vi "AddVIsToDictionary.vi"(7 "VIs in":refnum<vi>[](array[refnum]), 8 "error in (no error)":errorcluster, 11 "Dictionary from File":T1) -> (0 "error out":errorcluster, 3 "Merged Dictionary":T1)   [LabVIEW 2017, in "JKI Simple Localization.lvlib"]
uses:
  API/JKI Simple Localization.lvlib
  Definitions/Dictionary--Cluster.ctl
  Definitions/Private/FontCluster.ctl
  Definitions/Private/Phrase Dictionary.ctl
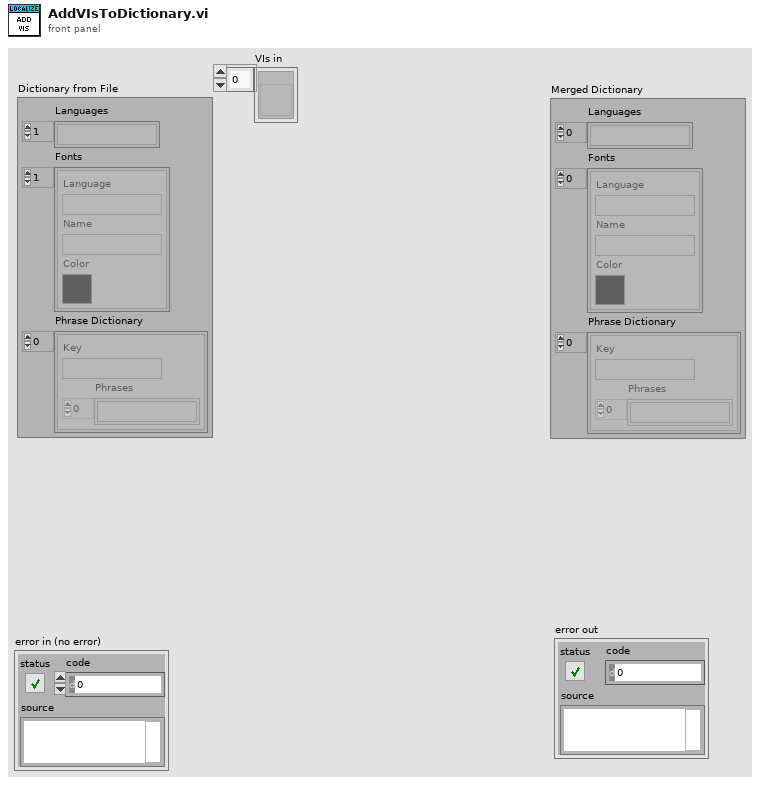
[diagram p1: front panel]
types:
  T1 = typedef "JKI Simple Localization.lvlib/Dictionary--Cluster.ctl" = cluster{"Languages":string[], "Fonts":T2[], "Phrase Dictionary":T3[]}
  T2 = typedef "JKI Simple Localization.lvlib/FontCluster.ctl" = cluster{"Language":string, "Name":string, "Color":u32}
  T3 = typedef "JKI Simple Localization.lvlib/Phrase Dictionary.ctl" = cluster{"Key":string, "Phrases":string[]}
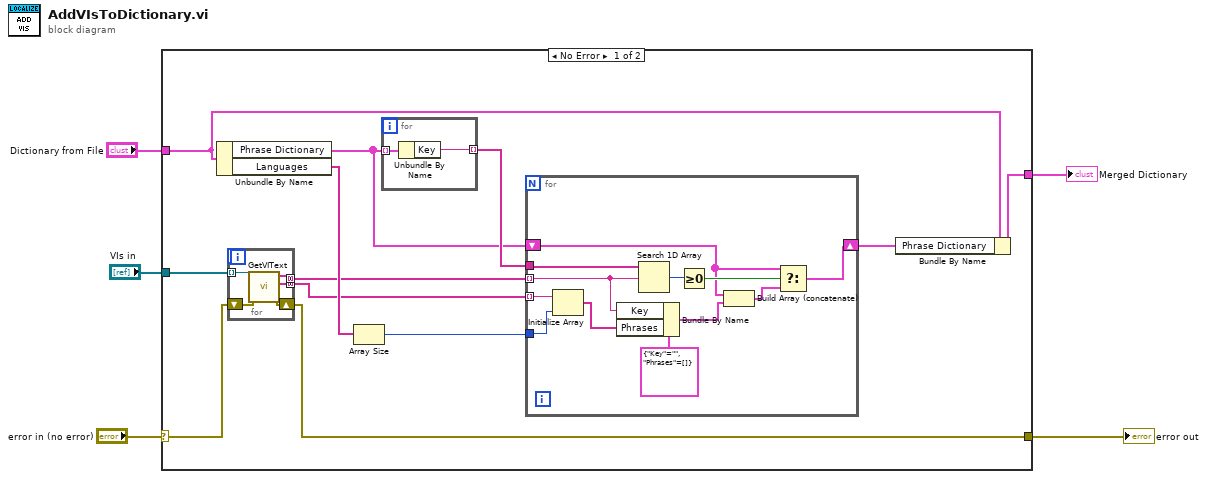
[diagram p0: block diagram]
diagram:
  n1 = case shown="No Error" "error in (no error)" {
    selector: "error in (no error)" -> [w14 w38]
    tunnel: [w13 w38] -> w4
    tunnel: "Dictionary from File" -> [w16 w37]
    tunnel: [w17 w37] -> w2
    tunnel: "VIs in" -> [w15 _]
    frame No Error {
      n2 = Unbundle By Name(w16) -> ("Phrase Dictionary"=w11:T3[], "Languages"=w10:string[])
      n3 = for {
        tunnel: [w22] -> w6 mode=concatenating
        tunnel: [w21] -> w7 mode=concatenating
        shift-right: [w20] -> w13
        shift-left: w14 -> [w19]
        tunnel: w15 -> [w18] mode=indexing
        n4 = call "GetVIText.vi"("error in (no error)"=w19, "VI"=w18) -> ("error out"=w20:errorcluster, "Control Text"=w22:string[], "Control Keys"=w21:string[])  [unwired: 7 in]
      }
      n5 = Array Size(array=w10) -> (size(s)=w9:i32)
      n6 = for {
        tunnel: w11 -> [w24] mode=indexing
        tunnel: [w23] -> w12 mode=indexing
        n7 = Unbundle By Name(w24) -> ("Key"=w23:string)
      }
      n8 = for {
        tunnel: w7 -> [w32] mode=indexing
        tunnel: w12 -> [w36]
        shift-right: [w25] -> w8
        shift-left: w11 -> [w28]
        tunnel: w6 -> [w31] mode=indexing
        tunnel: w9 -> [w30]
        n9 = Initialize Array(w31, w30) -> (w29:string[])
        n10 = Bundle By Name(cluster=T3 {"Key"="", "Phrases"=[]} ("input cluster"), "Key"=w32, "Phrases"=w29) -> (w27:T3)
        n11 = Search 1D Array(1D array=w36, element=w32) -> (index of element=w35:i32)  [unwired: 1 in]
        n12 = Greater Or Equal To 0?(x=w35) -> (x >= 0?=w34:bool)
        n13 = Build Array (concatenate)(w28, w27) -> (w26:T3[])
        n14 = Select(t=w28, s=w34, f=w26) -> (s? t:f=w25:T3[])
      }
      n15 = Bundle By Name(cluster=w16, "Phrase Dictionary"=w8) -> (w17:T1)
    }
    frame Error {
    }
  }
  "error out" <- w4
  "Merged Dictionary" <- w2
